vi "TechnosoftDecodeReturn.vi"(0 "expect return":T1(ring), 1 "unsigned byte array in":u8[](array[numeric])=[15, 241, 180, 5, 15, 240, 2, 178, 126, 64, 0, 5, 59] format="%02x", 2 "error in (no error)":errorcluster) -> (3 "comment":string, 4 "name":string, 5 "Value":dbl=360000.0, 6 "error out":errorcluster)   [LabVIEW 2011]
panel:
  out "checksum":bool=TRUE
  out "Address":u16=690 format="%x"
  out "Axis":u16=4080 format="%x"
  out "u16 data":u16[](array[numeric])=[4081, 46085, 4080, 690, 32320, 5] format="%04x"
  out "checksum":u8=59 format="%x"
  out "sum":u8=59 format="%x"
  # "axis"
  # "value"
  # "relayaxis"
  # "Parameter?"
  # "if B404 (16bit) or B405 (32bit) from SRAM data, or SRAM prog, or EEPROM"
  # "format unknown to: @0xFFFF"
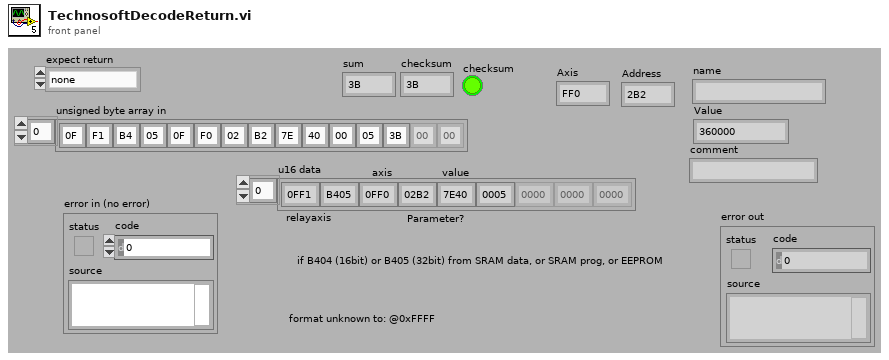
[diagram p1: front panel]
types:
  T1 = enum8{"none", "program32", "program16", "data32", "data16", "eprom32", "eprom16", "somethingelse32", "somethingelse16"}
  T2 = cluster{string[], u32[], enum16{"unknown", "i16", "u16", "i32", "u32", "fix32"}[], "comment":string[]}
  T3 = enum16{"unknown", "i16", "u16", "i32", "u32", "fix32"}[]
  T4 = enum16{"unknown", "i16", "u16", "i32", "u32", "fix32"}
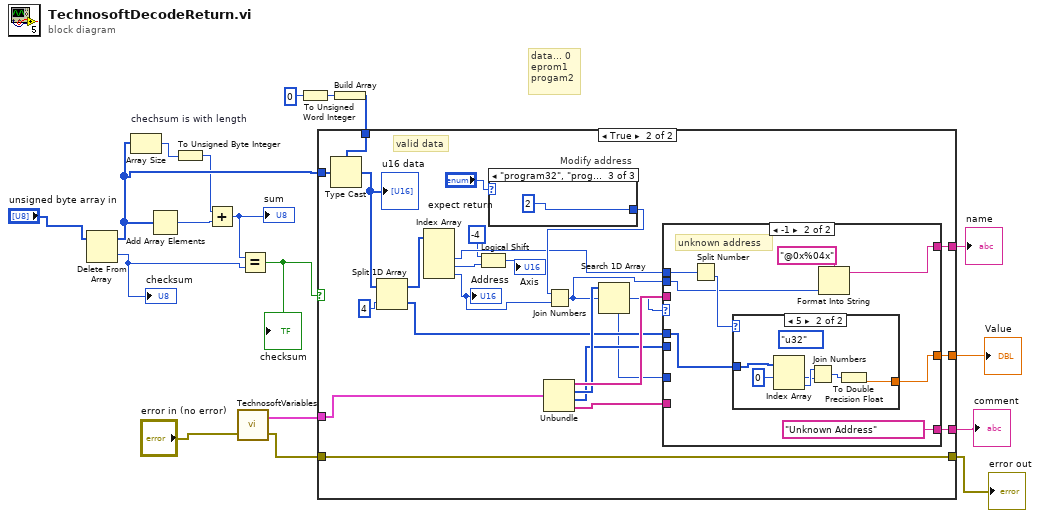
[diagram p0: block diagram]
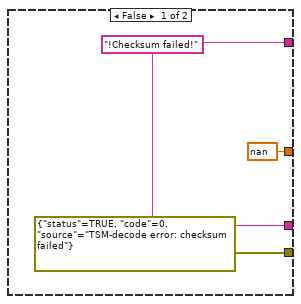
[diagram p2: hidden frame]
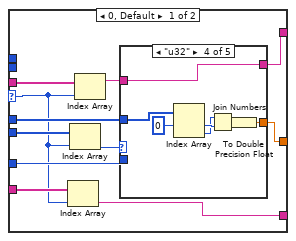
[diagram p3: hidden frame]
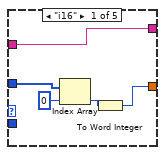
[diagram p4: hidden frame]
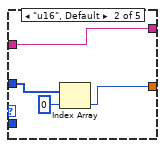
[diagram p5: hidden frame]
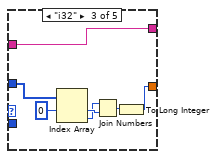
[diagram p6: hidden frame]
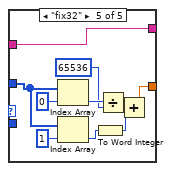
[diagram p7: hidden frame]
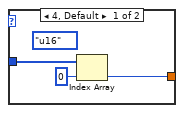
[diagram p8: hidden frame]
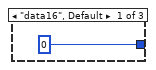
[diagram p9: hidden frame]
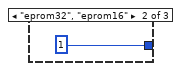
[diagram p10: hidden frame]
diagram:
  # "data... 0\neprom1\nprogam2"
  n1 = Delete From Array(array="unsigned byte array in") -> (deleted portion=w14:u8, array with subset deleted=w12:u8[])  [unwired: 2 in]
  "checksum" <- w14
  n2 = Array Size "chechsum is with length"(array=w12) -> (size(s)=w16:i32)
  n3 = Add Array Elements(numeric array=w12) -> (sum=w18:u8)
  n4 = To Unsigned Byte Integer(number=w16) -> (unsigned 8bit integer=w6:u8)
  n5 = Add(x=w6, y=w18) -> (x+y=w15:u8)
  "sum" <- w15
  n6 = call "TechnosoftVariables.vi"("error in (no error)"="error in (no error)") -> ("error out"=w1:errorcluster, "TSM variable table"=w3:T2)  [unwired: 2 out]
  n7 = Equal?(x=w15, y=w14) -> (x = y?=w13:bool)
  "checksum" <- w13
  n8 = To Unsigned Word Integer(number=0) -> (unsigned 16bit integer=w10:u16)
  n9 = Build Array(w10) -> (w9:u16[])
  n10 = case shown="True" w13 {
    tunnel: w12 -> [_ w44]
    tunnel: w9 -> [_ w43]
    tunnel: [nan w42] -> w8
    tunnel: [w20 w34] -> w7
    tunnel: [w20 w41] -> w5
    tunnel: w1 -> [_ w40]
    tunnel: [errorcluster {"status"=TRUE, "code"=0, "source"="TSM-decode error: checksum failed"} ("error in (no error)") w40] -> w4
    tunnel: w3 -> [_ w39]
    frame False {
      w20 = "!Checksum failed!" ("name")
    }
    frame True {
      # "valid data"
      n11 = Type Cast(type=w43, x=w44) -> (*(type *) &x=w33:u16[])
      "u16 data" <- w33
      n12 = Split 1D Array(array=w33, index=4) -> (first subarray=w32:u16[], second subarray=w31:u16[])
      n13 = Index Array(array=w32) -> (element #2=w26:u16, element #3=w24:u16, element #4=w30:u16)  [unwired: 4 in, 1 out]
      "Address" <- w30
      n14 = Logical Shift(y=i8 -4, x=w24) -> (x << y=→"Axis":u16)
      n15 = case "Modify address" shown="\"program32\", \"program16\"" "expect return" {
        tunnel: [u16 0 ("hi") u16 1 ("hi") u16 2 ("hi")] -> w28
        frame "data16", Default {
        }
        frame "eprom32", "eprom16" {
        }
        frame "program32", "program16" {
        }
      }
      n16 = Unbundle(w39) -> (w38:string[], w37:u32[], w36:T3, "comment"=w35:string[])
      n17 = Join Numbers(hi=w28, lo=w30) -> ((hi.lo)=w25:u32)
      n18 = Search 1D Array(1D array=w37, element=w25) -> (index of element=w27:i32)  [unwired: 1 out]
      n19 = case shown="-1" w27 {
        selector: w27 -> [w46 _]
        tunnel: [w55 w91] -> w42
        tunnel: [w54 "Unknown Address" ("comment")] -> w41
        tunnel: w38 -> [w53 _]
        tunnel: w36 -> [w52 _]
        tunnel: w35 -> [w51 _]
        tunnel: [w49 w92] -> w34
        tunnel: w31 -> [w48 w95]
        tunnel: w25 -> [w47 _]
        tunnel: w26 -> [_ w96]
        tunnel: w25 -> [_ w94]
        frame 0, Default {
          n20 = Index Array(array=w51, index=w46) -> (element=w54:string)
          n21 = Index Array(array=w52, index=w46) -> (element=w56:T4)
          n22 = Index Array(array=w53, index=w46) -> (element=w50:string)
          n23 = case shown="\"u32\"" w56 {
            tunnel: w48 -> [w60 w64 w70 w77 w87]
            tunnel: [w58 w63 w68 w75 w83] -> w55
            tunnel: w47 -> [_ _ _ _ _]
            tunnel: w50 -> [w57 w62 w67 w74 w80]
            tunnel: [w57 w62 w67 w74 w80] -> w49
            frame "i16" {
              n24 = Index Array(array=w60, index=0) -> (element=w59:u16)
              n25 = To Word Integer(number=w59) -> (16bit integer=w58:i16)
            }
            frame "u16", Default {
              n26 = Index Array(array=w64, index=0) -> (element=w63:u16)
            }
            frame "i32" {
              n27 = Index Array(array=w70, index #1=0 ("index")) -> (element #1=w72:u16, element #2=w66:u16)  [unwired: 1 in]
              n28 = Join Numbers(hi=w66, lo=w72) -> ((hi.lo)=w69:u32)
              n29 = To Long Integer(number=w69) -> (32bit integer=w68:i32)
            }
            frame "u32" {
              n30 = Index Array(array=w77, index #1=0 ("index")) -> (element #1=w79:u16, element #2=w73:u16)  [unwired: 1 in]
              n31 = Join Numbers(hi=w73, lo=w79) -> ((hi.lo)=w76:u32)
              n32 = To Double Precision Float(number=w76) -> (double precision float=w75:dbl)
            }
            frame "fix32" {
              n33 = Index Array(array=w87, index=0) -> (element=w86:u16)
              n34 = Index Array(array=w87, index=1) -> (element=w85:u16)
              n35 = To Word Integer(number=w85) -> (16bit integer=w81:i16)
              n36 = Divide(x=w86, y=65536) -> (x/y=w84:dbl)
              n37 = Add(x=w84, y=w81) -> (x+y=w83:dbl)
            }
          }
        }
        frame -1 {
          # "unknown address"
          n38 = Split Number(x=w96) -> (lo(x)=w97:u8)  [unwired: 1 out]
          n39 = case shown="5" w97 {
            tunnel: w95 -> [w99 w102]
            tunnel: [w98 w101] -> w91
            frame 4, Default {
              (unwired) T4."u16" ("element")
              n40 = Index Array(array=w99, index=0) -> (element=w98:u16)
            }
            frame 5 {
              (unwired) T4."u32" ("element")
              n41 = Index Array(array=w102, index #1=0 ("index")) -> (element #1=w103:u16, element #2=w106:u16)  [unwired: 1 in]
              n42 = Join Numbers(hi=w106, lo=w103) -> ((hi.lo)=w105:u32)
              n43 = To Double Precision Float(number=w105) -> (double precision float=w101:dbl)
            }
          }
          n44 = Format Into String(format string="@0x%04x", w94) -> (resulting string=w92:string)  [unwired: 2 in, 1 out]
        }
      }
    }
  }
  "Value" <- w8
  "name" <- w7
  "comment" <- w5
  "error out" <- w4
